vi "Alltesta Test.vi"() -> ()   [LabVIEW 2023, in "Alltesta Autosampler.lvlib"]
uses:
  Alltesta Autosampler.lvlib
panel:
  in  "Shake Trak":bool
  in  "Wash Needle":bool
  in  "Move Pos":dbl min=0.0 max=5004.0 step=1.0 format="%#_13g"
  in  "Move Tray":bool
  in  "Fill Vol":dbl min=0.0 max=120.0 step=1.0 format="%#_13g"
  in  "Set Fill":bool
  in  "Valve Index":dbl=1.0 min=1.0 max=6.0 step=1.0 format="%#_13g"
  in  "Set Valve":bool
  in  "Lower Needle":bool
  in  "Raise Needle":bool
  out "error out":errorcluster
  in  "Exit":bool
  in  "Send":bool
  in  "Command":string
  out "Response":string
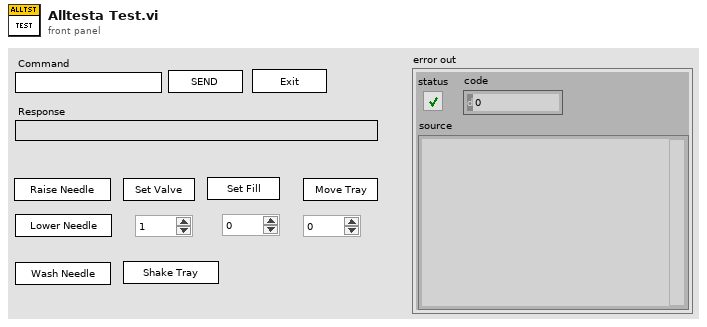
[diagram p1: front panel]
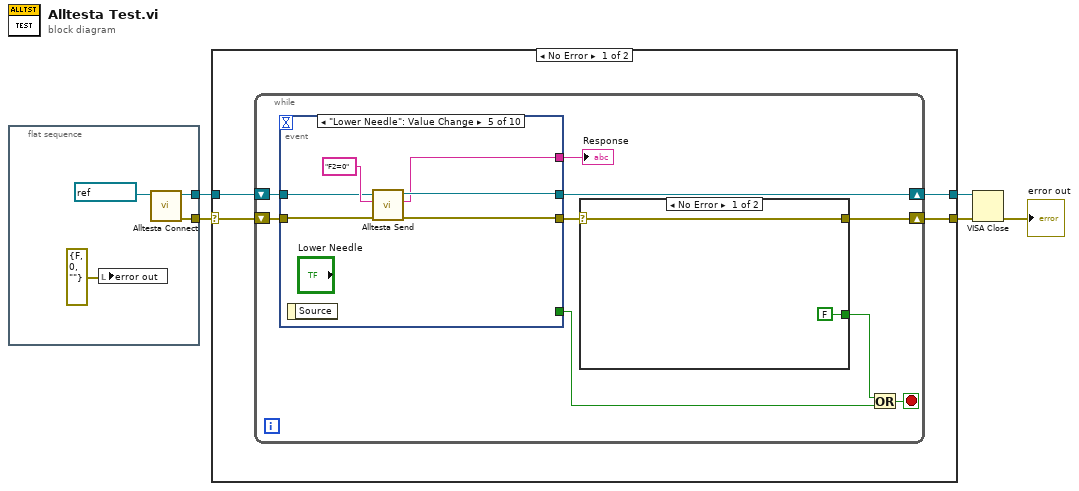
[diagram p0: block diagram]
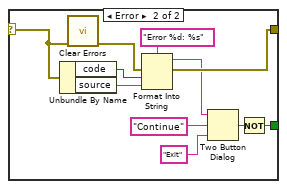
[diagram p2: hidden frame]
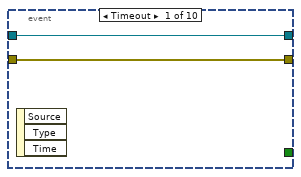
[diagram p3: hidden frame]
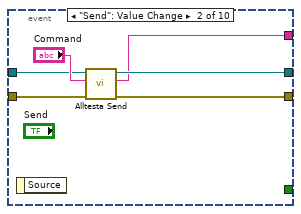
[diagram p4: hidden frame]
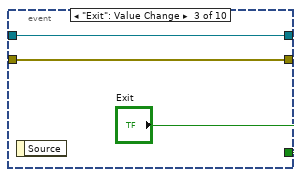
[diagram p5: hidden frame]
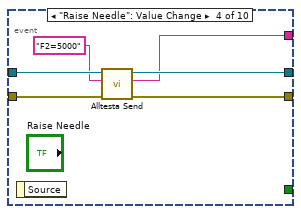
[diagram p6: hidden frame]
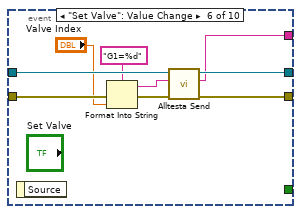
[diagram p7: hidden frame]
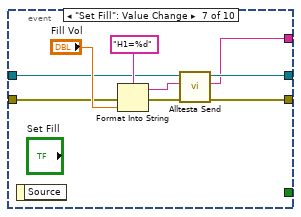
[diagram p8: hidden frame]
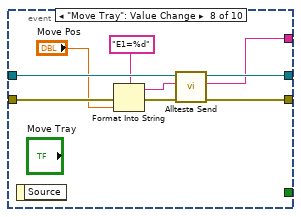
[diagram p9: hidden frame]
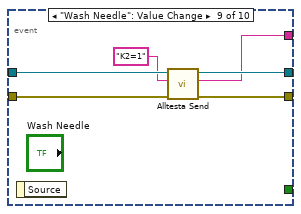
[diagram p10: hidden frame]
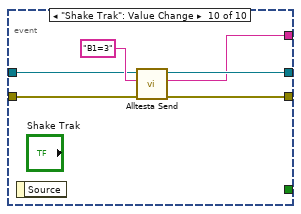
[diagram p11: hidden frame]
diagram:
  n1 = flat-sequence {
    tunnel: [w8] -> w5
    tunnel: [w7] -> w1
    frame #0 {
      n2 = local write "error out"(errorcluster {"status"=FALSE, "code"=0, "source"=""} ("error constant")) -> ()
      n3 = call "Alltesta Connect.vi"("VISA resource name"=refnum<visa-resource-name> "COM5") -> ("error out"=w7:errorcluster, "VISA resource name out"=w8:refnum<visa-resource-name>)  [unwired: 9 in]
    }
  }
  n4 = case shown="No Error" w1 {
    selector: w1 -> [w10 w98]
    tunnel: w5 -> [w13 w99]
    tunnel: [w12 w99] -> w4
    tunnel: [w11 w98] -> w3
    frame No Error {
      n5 = while {
        shift-right: [w18] -> w11
        shift-left: w10 -> [w22]
        shift-right: [w20] -> w12
        shift-left: w13 -> [w21]
        stop <- w17 stop-if-true
        n6 = event shown="[4] \"Lower Needle\": Value Change" {
          selector: _ -> [_ _ _ _ _ _ _ _ _ _]
          dyn-events: _ -> [_ _ _ _ _ _ _ _ _ _]
          timeout: _ -> [_ _ _ _ _ _ _ _ _ _]
          tunnel: w22 -> [w36 w41 w45 w51 w56 w64 w72 w80 w91 w96]
          tunnel: w21 -> [w37 w42 w46 w52 w57 w67 w70 w83 w87 w92]
          tunnel: [w37 w40 w46 w49 w54 w65 w69 w82 w89 w94] -> w20
          tunnel: [w36 w39 w45 w50 w55 w66 w71 w81 w90 w95] -> w19
          tunnel: [_ _ "Exit" _ _ _ _ _ _ _] -> w15
          tunnel: [_ w38 _ w47 w53 w59 w68 w79 w88 w93] -> w14
          event Timeout {
            n7 = event-data() -> ()  [unwired: 1 in, 3 out]
          }
          event "Send": Value Change {
            n8 = event-data() -> ()  [unwired: 1 in, 1 out]
            n9 = call "Alltesta Send.vi"("error in (no error)"=w41, "Command"="Command", "Serial Port in"=w42) -> ("error out"=w39:errorcluster, "Response"=w38:string, "Serial Port out"=w40:refnum<visa-resource-name>)  [unwired: 6 in]
          }
          event "Exit": Value Change {
            n10 = event-data() -> ()  [unwired: 1 in, 1 out]
          }
          event "Raise Needle": Value Change {
            n11 = event-data() -> ()  [unwired: 1 in, 1 out]
            n12 = call "Alltesta Send.vi"("error in (no error)"=w51, "Command"="F2=5000", "Serial Port in"=w52) -> ("error out"=w50:errorcluster, "Response"=w47:string, "Serial Port out"=w49:refnum<visa-resource-name>)  [unwired: 6 in]
          }
          event "Lower Needle": Value Change {
            n13 = event-data() -> ()  [unwired: 1 in, 1 out]
            n14 = call "Alltesta Send.vi"("error in (no error)"=w56, "Command"="F2=0", "Serial Port in"=w57) -> ("error out"=w55:errorcluster, "Response"=w53:string, "Serial Port out"=w54:refnum<visa-resource-name>)  [unwired: 6 in]
          }
          event "Set Valve": Value Change {
            n15 = event-data() -> ()  [unwired: 1 in, 1 out]
            n16 = Format Into String(format string="G1=%d", error in=w64, "Valve Index") -> (resulting string=w61:string, error out=w63:errorcluster)  [unwired: 1 in]
            n17 = call "Alltesta Send.vi"("error in (no error)"=w63, "Command"=w61, "Serial Port in"=w67) -> ("error out"=w66:errorcluster, "Response"=w59:string, "Serial Port out"=w65:refnum<visa-resource-name>)  [unwired: 6 in]
          }
          event "Set Fill": Value Change {
            n18 = event-data() -> ()  [unwired: 1 in, 1 out]
            n19 = Format Into String(format string="H1=%d", error in=w72, "Fill Vol") -> (resulting string=w75:string, error out=w76:errorcluster)  [unwired: 1 in]
            n20 = call "Alltesta Send.vi"("error in (no error)"=w76, "Command"=w75, "Serial Port in"=w70) -> ("error out"=w71:errorcluster, "Response"=w68:string, "Serial Port out"=w69:refnum<visa-resource-name>)  [unwired: 6 in]
          }
          event "Move Tray": Value Change {
            n21 = event-data() -> ()  [unwired: 1 in, 1 out]
            n22 = Format Into String(format string="E1=%d", error in=w80, "Move Pos") -> (resulting string=w84:string, error out=w85:errorcluster)  [unwired: 1 in]
            n23 = call "Alltesta Send.vi"("error in (no error)"=w85, "Command"=w84, "Serial Port in"=w83) -> ("error out"=w81:errorcluster, "Response"=w79:string, "Serial Port out"=w82:refnum<visa-resource-name>)  [unwired: 6 in]
          }
          event "Wash Needle": Value Change {
            n24 = event-data() -> ()  [unwired: 1 in, 1 out]
            n25 = call "Alltesta Send.vi"("error in (no error)"=w91, "Command"="K2=1", "Serial Port in"=w87) -> ("error out"=w90:errorcluster, "Response"=w88:string, "Serial Port out"=w89:refnum<visa-resource-name>)  [unwired: 6 in]
          }
          event "Shake Trak": Value Change {
            n26 = event-data() -> ()  [unwired: 1 in, 1 out]
            n27 = call "Alltesta Send.vi"("error in (no error)"=w96, "Command"="B1=3", "Serial Port in"=w92) -> ("error out"=w95:errorcluster, "Response"=w93:string, "Serial Port out"=w94:refnum<visa-resource-name>)  [unwired: 6 in]
          }
        }
        "Response" <- w14
        n28 = case shown="No Error" w19 {
          selector: w19 -> [w24 w25]
          tunnel: [FALSE w33] -> w16
          tunnel: [w24 w28] -> w18
          frame No Error {
          }
          frame Error {
            n29 = Unbundle By Name(w25) -> ("code"=w31:i32, "source"=w30:string)
            n30 = call <vilib>:"Clear Errors.vi"("error in (no error)"=w25) -> ("error out"=w29:errorcluster)  [unwired: 5 in, 1 out]
            n31 = Format Into String(format string="Error %d: %s", error in=w29, w31, w30) -> (resulting string=w27:string, error out=w28:errorcluster)  [unwired: 1 in]
            n32 = Two Button Dialog(message=w27, 1:"Exit" ("F button name (\"Cancel\")"), 2:"Continue" ("T button name (\"OK\")")) -> (T button?=w32:bool)
            n33 = Not(x=w32) -> (.not. x?=w33:bool)
          }
        }
        n34 = Or(x=w16, y=w15) -> (x .or. y?=w17:bool)
      }
    }
    frame Error {
    }
  }
  n35 = VISA Close(VISA resource name=w4, error in (no error)=w3) -> (error out=→"error out":errorcluster)
